vi "Autonomous Independent.vi"() -> ()   [LabVIEW 2014]
doc: "This VI is called when autonomous begins, and will automatically be terminated when autonomous ends. You can carry out timed or sensor driven robot movement independently without needing to return to the caller."
uses:
  <vilib>/Rock Robotics/WPI/SafetyOutput/WPI_SafetyOutputConfigMenu.ctl
  <vilib>/Rock Robotics/WPI/Joystick/WPI_JoystickGetSetRefNum.vi
  <vilib>/Rock Robotics/Network Tables/SD Read Boolean.vi
  <vilib>/Rock Robotics/Network Tables/SD Write Boolean.vi
  AutoVar.vi
  <vilib>/Rock Robotics/WPI/RobotDrive/WPI_RobotDriveGetSetRefNum.vi
  Global 2.vi
  <vilib>/Rock Robotics/WPI/RobotDrive/WPI_RobotDriveArcadeDrive_Standard(NoSaturation).vi
panel:
  out "Boolean1 2":bool
  out "Boolean1 3":bool
  out "Boolean1":bool
  out "Current Movement, for debugging":T1 {"Y Joystick Value" scale=1.0..-1.0; "X Joystick Value" scale=-1.0..1.0}
  in  "Array of robot movements":T2(array[cluster]) {"Y Joystick Value" scale=1.0..-1.0; "X Joystick Value" scale=-1.0..1.0}
  # "Be sure to right-click and choose Data Operations>>Make Current Value default if you want to save the array values with the VI"
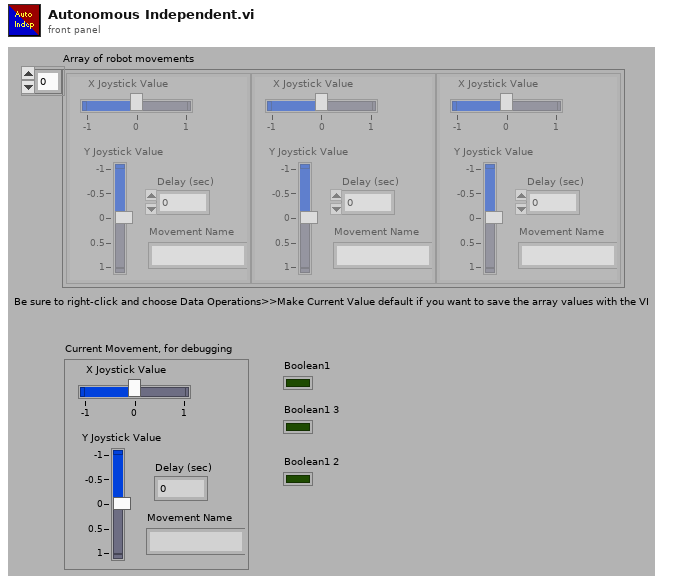
[diagram p1: front panel]
types:
  T1 = cluster{"X Joystick Value":dbl, "Y Joystick Value":dbl, "Delay (sec)":dbl, "Movement Name":string}
  T2 = cluster{"X Joystick Value":dbl, "Y Joystick Value":dbl, "Delay (sec)":dbl, "Movement Name":string}[]
  T3 = typedef "WPI_SafetyOutputConfigMenu.ctl" = enum16{"Enable", "Disable"}
  T4 = typedef "WPI_MotorControlDeviceRef.ctl" = cluster{"DeviceStatus":errorcluster, "Type":T5, "PWM":cluster{"Controller":T6, "PWM Channel":T7, "DeadBand":T8}, "CAN":cluster{"Device Number":u8, "Control Mode":T9, "Semaphore":T10, "Max Vout":dbl, "TalonSRX Control Mode":T11}, "Invert":bool, "TransformRef":T12, "InvTransformRef":T12}
  T5 = typedef "WPI_MotorControlType.ctl" = enum16{"PWM", "CAN", "CANTalonSRX"}
  T6 = typedef "FPGA_TypedefDigitalModule.ctl" = enum16{"Controller 1"}
  T7 = typedef "FPGA_DIOPWMChannel.ctl" = enum8{"PWM 0", "PWM 1", "PWM 2", "PWM 3", "PWM 4", "PWM 5", "PWM 6", "PWM 7", "PWM 8", "PWM 9", "PWM MXP 0", "PWM MXP 1", "PWM MXP 2", "PWM MXP 3", "PWM MXP 4", "PWM MXP 5", "PWM MXP 6", "PWM MXP 7", "PWM MXP 8", "PWM MXP 9", "Invalid"}
  T8 = typedef "WPI_PWMDeadband.ctl" = cluster{"Name":string, "maxPositivePwm":i32, "minPositivePwm":i32, "centerPwm":i32, "maxNegativePwm":i32, "minNegativePwm":i32, "angularRange":u16}
  T9 = typedef "WPI_CANJaguar_ControlMode.ctl" = enum8{"Percent VBus", "Current", "Speed", "Position", "Voltage"}
  T10 = typedef "Semaphore RefNum" = refnum<k1>
  T11 = typedef "WPI_CANTalonSRX_APIControlMode.ctl" = enum8{"Percent VBus", "Speed", "Position", "Slave", "Unchanged / Invalid"}
  T12 = typedef "WPI_PWMTransform_ConPane.ctl" = refnum<vi>
  T13 = typedef "WPI_RobotDriveDevRef.ctl" = cluster{"DevStatus":errorcluster, "Motors[]":T4[], "Square Inputs":bool, "Max Output":dbl}
  T14 = typedef "WPI_JoystickDevRef.ctl" = cluster{"Device":T15}
  T15 = typedef "WPI_JoystickDeviceEnum.ctl" = enum16{"USB 0", "USB 1", "USB 2", "USB 3", "USB 4", "USB 5"}
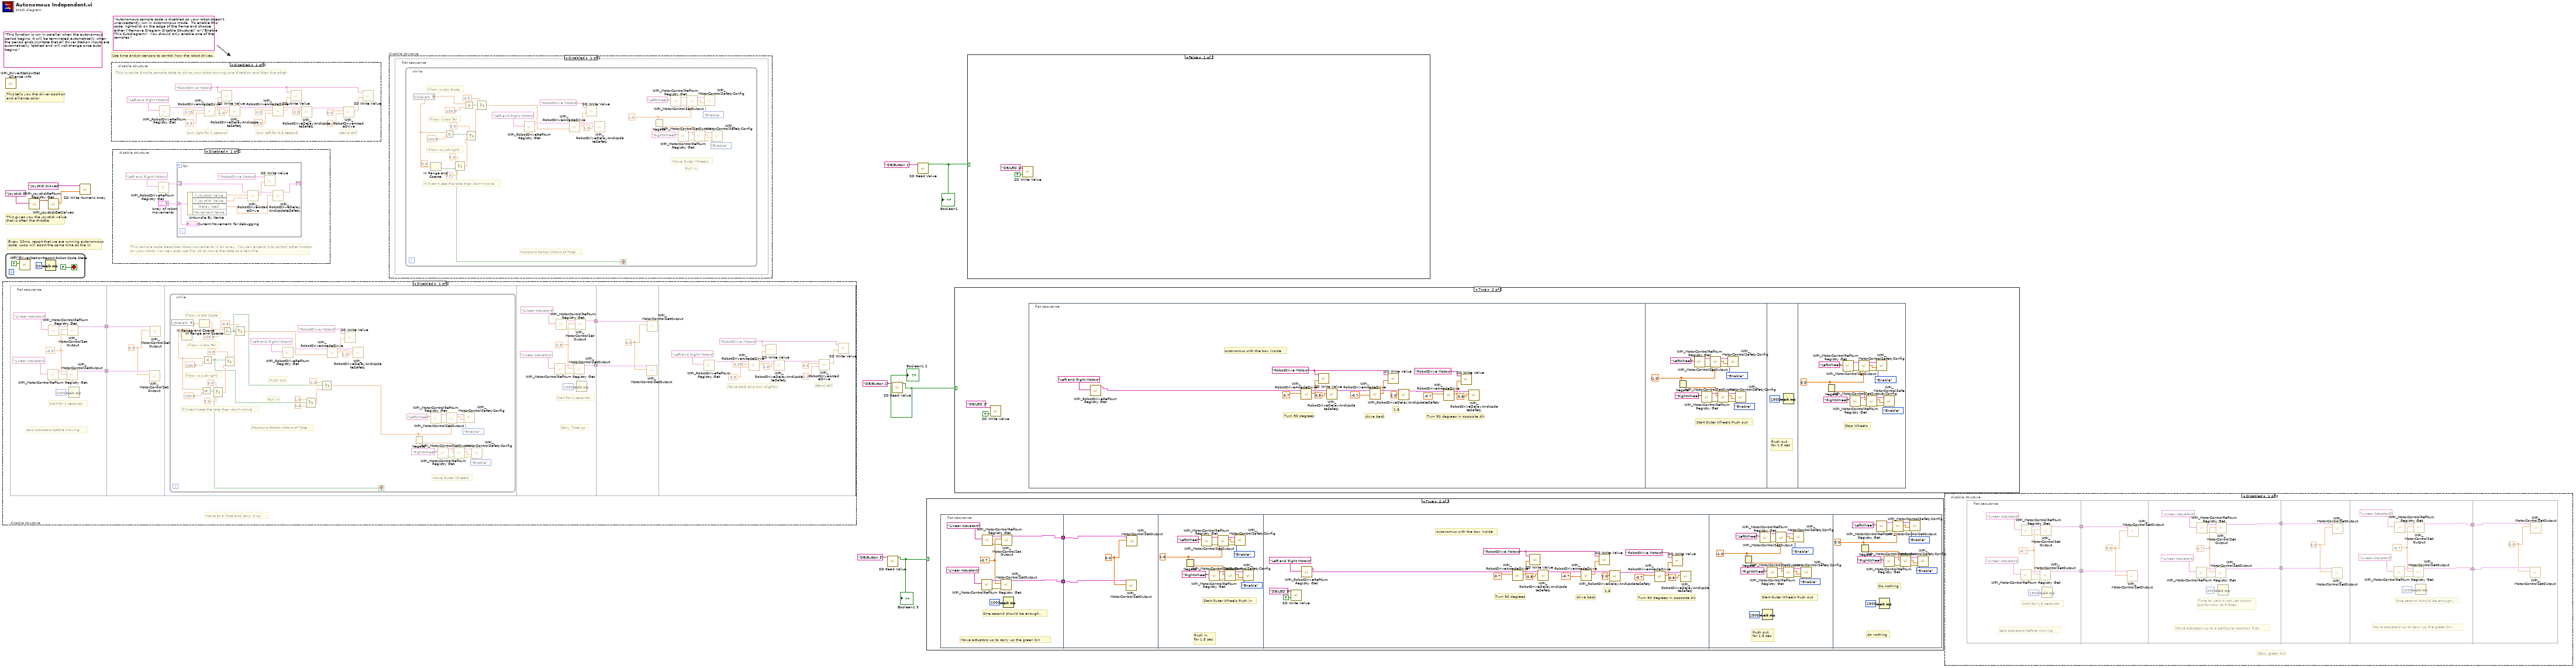
[diagram p0: block diagram]
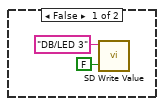
[diagram p3: hidden frame]
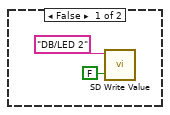
[diagram p4: hidden frame]
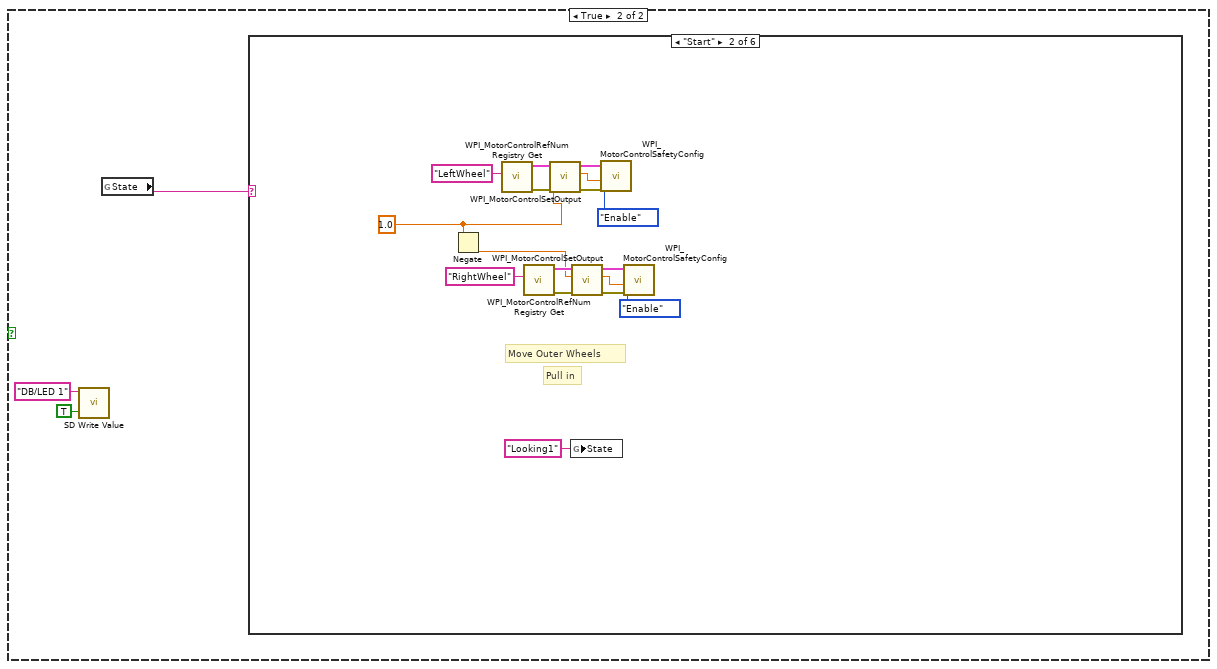
[diagram p5: hidden frame]
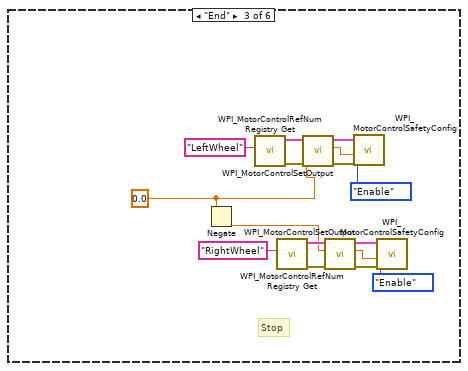
[diagram p7: hidden frame]
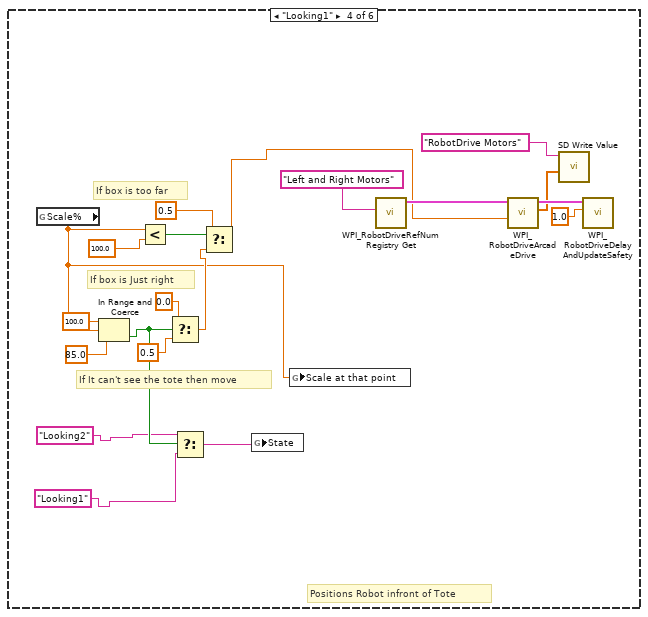
[diagram p8: hidden frame]
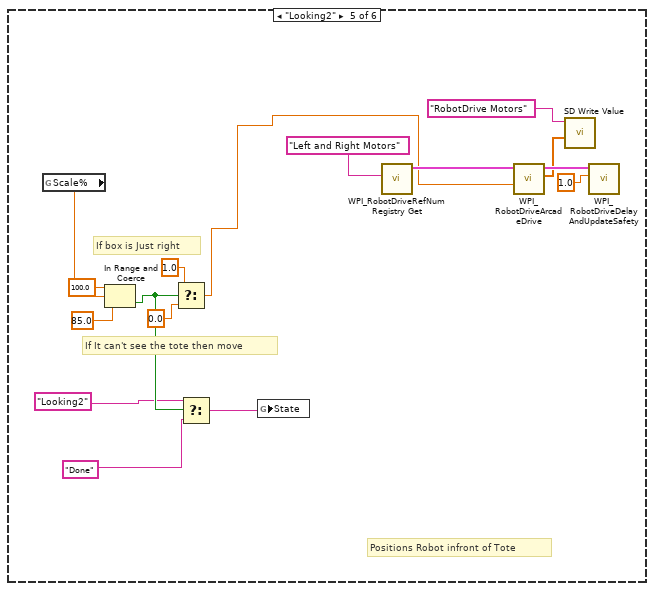
[diagram p9: hidden frame]
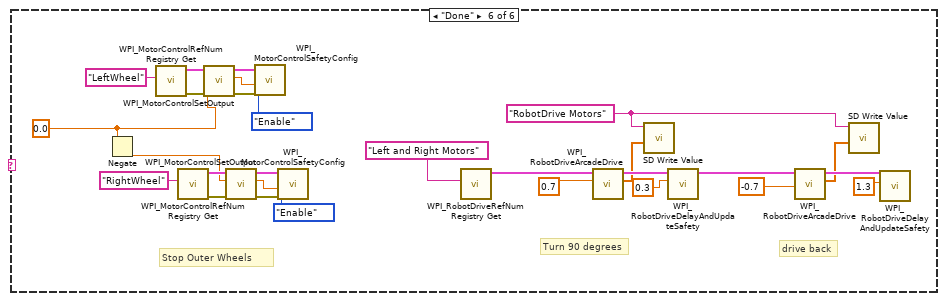
[diagram p10: hidden frame]
diagram:
  (unwired) "Autonomous sample code is disabled so your robot doesn't unexpectantly run in Autonomous mode.  To enable this code, right-click on the edge of the frame and choose either \"Remove Diagram Disable Structure\" or \"Enable This Subdiagram\". You should only enable one of the samples."
  (unwired) "This function is run in parallel when the autonomous period begins. It will be terminated automatically when the period ends.\n\nNote that all Driver Station inputs are automatically latched and will not change once auto begins."
  # "Every 20ms, report that we are running autonomous\ncode. Loop will abort the same time as the VI."
  # "This gives you the joystick value\nthat is often the throttle"
  # "Use time and/or sensors to control how the robot drives."
  # "This tells you the driver position\nand alliance color"
  n1 = disable-structure shown="Disabled" {
    frame Disabled {
      # "Move to a Tote and carry it up"
      n2 = flat-sequence {
        tunnel: [w16] -> w14
        tunnel: [w15] -> w13
        tunnel: w14 -> [w27]
        tunnel: w13 -> [w26]
        tunnel: [w71] -> w12
        tunnel: [w70] -> w11
        tunnel: w12 -> [w81]
        tunnel: w11 -> [w80]
        frame #0 {
          w18 = -0.5 ("Output")
          # "zero actuators before moving"
          # "Wait for 1 seconds"
          n3 = call <vilib>:"WPI_MotorControlRefNum Registry Get.vi"("refnum name"="Linear Actuator1") -> ("error out"=w21:errorcluster, "MotorControlDevRef"=w20:T4)  [unwired: 9 in]
          n4 = call <vilib>:"WPI_MotorControlRefNum Registry Get.vi"("refnum name"="Linear Actuator0") -> ("error out"=w24:errorcluster, "MotorControlDevRef"=w23:T4)  [unwired: 9 in]
          n5 = call <vilib>:"WPI_MotorControlSetOutput.vi"("error in (no error)"=w21, "Output"=w18, "MotorControlDevRef"=w20) -> ("MotorControlDevRef"=w15:T4)  [unwired: 6 in, 2 out]
          n6 = call <vilib>:"WPI_MotorControlSetOutput.vi"("error in (no error)"=w24, "Output"=w18, "MotorControlDevRef"=w23) -> ("MotorControlDevRef"=w16:T4)  [unwired: 6 in, 2 out]
          n7 = Wait (ms)(milliseconds to wait=u32 1000) -> ()  [unwired: 1 out]
        }
        frame #1 {
          w25 = 0.0 ("Output")
          n8 = call <vilib>:"WPI_MotorControlSetOutput.vi"("Output"=w25, "MotorControlDevRef"=w26) -> ()  [unwired: 7 in, 3 out]
          n9 = call <vilib>:"WPI_MotorControlSetOutput.vi"("Output"=w25, "MotorControlDevRef"=w27) -> ()  [unwired: 7 in, 3 out]
        }
        frame #2 {
          n10 = while {
            stop <- w54 stop-if-true
            # "Move Outer Wheels"
            # "Pull in"
            # "Push out"
            # "If It can't see the tote then don't move"
            # "Positions Robot infront of Tote"
            # "If box is Just right"
            # "If box is too Far"
            # "If box is too close"
            n11 = global read "Global 2.vi" "Scale%"() -> (w29:dbl)
            n12 = In Range and Coerce(x=w29) -> (coerced(x)=w28:dbl)  [unwired: 2 in, 1 out]
            n13 = In Range and Coerce(x=w29) -> (coerced(x)=w30:dbl)  [unwired: 2 in, 1 out]
            n14 = Equal?(x=w28, y=100.0) -> (x = y?=w54:bool)
            n15 = Less?(x=w28, y=100.0) -> (x < y?=w33:bool)
            n16 = Select(t=0.0, s=w54, f=0.0) -> (s? t:f=w62:dbl)
            n17 = Greater?(x=w30, y=100.0) -> (0:w38:bool)
            n18 = Select(t=0.5, s=w33, f=w62) -> (s? t:f=w65:dbl)
            n19 = Select(t=-0.5, s=w38, f=w65) -> (s? t:f=w55:dbl)
            n20 = call <vilib>:"WPI_RobotDriveRefNum Registry Get.vi"("refnum name"="Left and Right Motors") -> ("RobotDriveDevRef"=w58:T13)  [unwired: 1 in, 9 out]
            n21 = Select(t=1.0, s=w33, f=0.0) -> (s? t:f=w34:dbl)
            n22 = Select(t=-1.0, s=w38, f=w34) -> (s? t:f=w36:dbl)
            n23 = call-poly <vilib>:"WPI_RobotDriveArcadeDrive.vi"("Y axis value"=w55, "RobotDriveDevRef"=w58) -> ("Motor Values"=w57:dbl[], "RobotDriveDevRef"=w61:T13)  [unwired: 2 in, 6 out]
            n24 = call-poly <vilib>:"SD Write Value.vi"("Numeric Array"=w57, "Name"="RobotDrive Motors") -> ()  [unwired: 8 in, 2 out]
            n25 = call <vilib>:"WPI_RobotDriveDelayAndUpdateSafety.vi"("Delay (s)"=1.0, "RobotDriveDevRef"=w61) -> ()  [unwired: 8 in, 2 out]
            n26 = Negate(x=w36) -> (-x=w35:dbl)
            n27 = call <vilib>:"WPI_MotorControlRefNum Registry Get.vi"("refnum name"="LeftWheel") -> ("error out"=w52:errorcluster, "MotorControlDevRef"=w51:T4)  [unwired: 9 in]
            n28 = call <vilib>:"WPI_MotorControlRefNum Registry Get.vi"("refnum name"="RightWheel") -> ("error out"=w50:errorcluster, "MotorControlDevRef"=w49:T4)  [unwired: 9 in]
            n29 = call <vilib>:"WPI_MotorControlSetOutput.vi"("error in (no error)"=w52, "Output"=w36, "MotorControlDevRef"=w51) -> ("error out"=w46:errorcluster, "Motor Output"=w45:dbl, "MotorControlDevRef"=w44:T4)  [unwired: 6 in]
            n30 = call <vilib>:"WPI_MotorControlSetOutput.vi"("error in (no error)"=w50, "Output"=w35, "MotorControlDevRef"=w49) -> ("error out"=w43:errorcluster, "Motor Output"=w42:dbl, "MotorControlDevRef"=w41:T4)  [unwired: 6 in]
            n31 = call <vilib>:"WPI_MotorControlSafetyConfig.vi"("error in (no error)"=w46, "timeout (s)"=w45, "mode"=WPI_SafetyOutputConfigMenu."Enable", "MotorControlDevRef"=w44) -> ()  [unwired: 6 in, 2 out]
            n32 = call <vilib>:"WPI_MotorControlSafetyConfig.vi"("error in (no error)"=w43, "timeout (s)"=w42, "mode"=WPI_SafetyOutputConfigMenu."Enable", "MotorControlDevRef"=w41) -> ()  [unwired: 6 in, 2 out]
          }
        }
        frame #3 {
          w73 = 0.5 ("Output")
          # "Carry Tote up"
          # "Wait for 1 seconds"
          n33 = call <vilib>:"WPI_MotorControlRefNum Registry Get.vi"("refnum name"="Linear Actuator1") -> ("error out"=w76:errorcluster, "MotorControlDevRef"=w75:T4)  [unwired: 9 in]
          n34 = call <vilib>:"WPI_MotorControlRefNum Registry Get.vi"("refnum name"="Linear Actuator0") -> ("error out"=w79:errorcluster, "MotorControlDevRef"=w78:T4)  [unwired: 9 in]
          n35 = call <vilib>:"WPI_MotorControlSetOutput.vi"("error in (no error)"=w76, "Output"=w73, "MotorControlDevRef"=w75) -> ("MotorControlDevRef"=w70:T4)  [unwired: 6 in, 2 out]
          n36 = call <vilib>:"WPI_MotorControlSetOutput.vi"("error in (no error)"=w79, "Output"=w73, "MotorControlDevRef"=w78) -> ("MotorControlDevRef"=w71:T4)  [unwired: 6 in, 2 out]
          n37 = Wait (ms)(milliseconds to wait=u32 1000) -> ()  [unwired: 1 out]
        }
        frame #4 {
          w82 = 0.0 ("Output")
          n38 = call <vilib>:"WPI_MotorControlSetOutput.vi"("Output"=w82, "MotorControlDevRef"=w80) -> ()  [unwired: 7 in, 3 out]
          n39 = call <vilib>:"WPI_MotorControlSetOutput.vi"("Output"=w82, "MotorControlDevRef"=w81) -> ()  [unwired: 7 in, 3 out]
        }
        frame #5 {
          w83 = "RobotDrive Motors" ("Name")
          # "stand still"
          # "Move back and turn slightly"
          n40 = call <vilib>:"WPI_RobotDriveRefNum Registry Get.vi"("refnum name"="Left and Right Motors") -> ("RobotDriveDevRef"=w90:T13)  [unwired: 1 in, 9 out]
          n41 = call-poly <vilib>:"WPI_RobotDriveArcadeDrive.vi"("Y axis value"=-0.5 ("X axis value"), "X axis value"=0.25, "RobotDriveDevRef"=w90) -> ("Motor Values"=w89:dbl[], "RobotDriveDevRef"=w93:T13)  [unwired: 1 in, 6 out]
          n42 = call-poly <vilib>:"SD Write Value.vi"("Numeric Array"=w89, "Name"=w83) -> ()  [unwired: 8 in, 2 out]
          n43 = call <vilib>:"WPI_RobotDriveDelayAndUpdateSafety.vi"("Delay (s)"=2.0, "RobotDriveDevRef"=w93) -> ("RobotDriveDevRef 2"=w84:T13)  [unwired: 8 in, 1 out]
          n44 = call-poly <vilib>:"WPI_RobotDriveArcadeDrive.vi"("Y axis value"=0.0 ("X axis value"), "X axis value"=0.0, "RobotDriveDevRef"=w84) -> ("Motor Values"=w85:dbl[])  [unwired: 1 in, 7 out]
          n45 = call-poly <vilib>:"SD Write Value.vi"("Numeric Array"=w85, "Name"=w83) -> ()  [unwired: 8 in, 2 out]
        }
      }
    }
    frame Enabled {
    }
  }
  n46 = while {
    stop <- FALSE stop-if-true
    n47 = call <vilib>:"WPI_DriverStationReport Robot Code State.vi"("Autonomous"=TRUE) -> ()  [unwired: 10 in, 1 out]
    n48 = Wait (ms)(milliseconds to wait=u32 20) -> ()  [unwired: 1 out]
  }
  n49 = call <vilib>:"WPI_DriverStationGet Alliance Info.vi"() -> ()  [unwired: 12 out]
  n50 = call <vilib>:"WPI_JoystickRefNum Registry Get.vi"("refnum name"="Joystick 0") -> ("JoystickDevRef"=w9:T14)  [unwired: 1 in, 9 out]
  n51 = call <vilib>:"WPI_JoystickGetValues.vi"("JoystickDevRef"=w9) -> ("Axes"=w7:dbl[])  [unwired: 6 in, 4 out]
  n52 = call <vilib>:"SD Write Numeric Array.vi"("Numeric Array"=w7, "Name"="Joystick 0/Axes") -> ()  [unwired: 8 in, 2 out]
  n53 = disable-structure shown="Disabled" {
    frame Disabled {
      w98 = "RobotDrive Motors" ("Name")
      # "This is some simple sample code to drive your robot curving one direction and then the other."
      # "stand still"
      # "turn left for 0.5 second"
      # "turn right for 1 second"
      n54 = call <vilib>:"WPI_RobotDriveRefNum Registry Get.vi"("refnum name"="Left and Right Motors") -> ("RobotDriveDevRef"=w102:T13)  [unwired: 1 in, 9 out]
      n55 = call-poly <vilib>:"WPI_RobotDriveArcadeDrive.vi"("Y axis value"=0.5 ("X axis value"), "X axis value"=0.25, "RobotDriveDevRef"=w102) -> ("Motor Values"=w101:dbl[], "RobotDriveDevRef"=w109:T13)  [unwired: 1 in, 6 out]
      n56 = call-poly <vilib>:"SD Write Value.vi"("Numeric Array"=w101, "Name"=w98) -> ()  [unwired: 8 in, 2 out]
      n57 = call <vilib>:"WPI_RobotDriveDelayAndUpdateSafety.vi"("Delay (s)"=1.0, "RobotDriveDevRef"=w109) -> ("RobotDriveDevRef 2"=w108:T13)  [unwired: 8 in, 1 out]
      n58 = call-poly <vilib>:"WPI_RobotDriveArcadeDrive.vi"("Y axis value"=0.25 ("X axis value"), "X axis value"=0.5, "RobotDriveDevRef"=w108) -> ("Motor Values"=w100:dbl[], "RobotDriveDevRef"=w107:T13)  [unwired: 1 in, 6 out]
      n59 = call-poly <vilib>:"SD Write Value.vi"("Numeric Array"=w100, "Name"=w98) -> ()  [unwired: 8 in, 2 out]
      n60 = call <vilib>:"WPI_RobotDriveDelayAndUpdateSafety.vi"("Delay (s)"=0.5, "RobotDriveDevRef"=w107) -> ("RobotDriveDevRef 2"=w106:T13)  [unwired: 8 in, 1 out]
      n61 = call-poly <vilib>:"WPI_RobotDriveArcadeDrive.vi"("Y axis value"=0.0 ("X axis value"), "X axis value"=0.0, "RobotDriveDevRef"=w106) -> ("Motor Values"=w99:dbl[])  [unwired: 1 in, 7 out]
      n62 = call-poly <vilib>:"SD Write Value.vi"("Numeric Array"=w99, "Name"=w98) -> ()  [unwired: 8 in, 2 out]
    }
    frame Enabled {
    }
  }
  n63 = disable-structure shown="Disabled" {
    frame Disabled {
      # "This sample code describes robot movements in an array. You can extend it to control other motors\non your robot. You can also use file I/O to move the data to a text file."
      n64 = call <vilib>:"WPI_RobotDriveRefNum Registry Get.vi"("refnum name"="Left and Right Motors") -> ("RobotDriveDevRef"=w117:T13)  [unwired: 1 in, 9 out]
      n65 = for {
        shift-right: [w125] -> _
        shift-left: w117 -> [w126]
        tunnel: "Array of robot movements" -> [w121] mode=indexing
        n66 = Unbundle By Name(w121) -> ("X Joystick Value"=w124:dbl, "Y Joystick Value"=w123:dbl, "Delay (sec)"=w122:dbl)  [unwired: 1 out]
        n67 = call-poly <vilib>:"WPI_RobotDriveArcadeDrive.vi"("Y axis value"=w123, "X axis value"=w124, "RobotDriveDevRef"=w126) -> ("Motor Values"=w119:dbl[], "RobotDriveDevRef"=w127:T13)  [unwired: 1 in, 6 out]
        n68 = call-poly <vilib>:"SD Write Value.vi"("Numeric Array"=w119, "Name"="RobotDrive Motors") -> ()  [unwired: 8 in, 2 out]
        n69 = call <vilib>:"WPI_RobotDriveDelayAndUpdateSafety.vi"("Delay (s)"=w122, "RobotDriveDevRef"=w127) -> ("RobotDriveDevRef 2"=w125:T13)  [unwired: 8 in, 1 out]
        "Current Movement, for debugging" <- w121
      }
    }
    frame Enabled {
    }
  }
  n70 = disable-structure shown="Disabled" {
    frame Disabled {
      n71 = flat-sequence {
        frame #0 {
          n72 = while {
            stop <- w131 stop-if-true
            w128 = 1.0 ("t")
            # "Move Outer Wheels"
            # "Pull in"
            # "If It can't see the tote then don't move"
            # "Positions Robot infront of Tote"
            # "If box is Just right"
            # "If box is too far"
            # "If box is too close"
            n73 = global read "Global 2.vi" "Scale%"() -> (w130:dbl)
            n74 = In Range and Coerce(upper limit=0.0, x=w130) -> (In Range?=w131:bool)  [unwired: 1 in, 1 out]
            n75 = Less?(x=w130, y=100.0) -> (x < y?=w132:bool)
            n76 = Select(t=0.0, s=w131, f=0.0) -> (s? t:f=w157:dbl)
            n77 = Greater?(x=w130, y=100.0) -> (0:w134:bool)
            n78 = Select(t=0.5, s=w132, f=w157) -> (s? t:f=w159:dbl)
            n79 = Select(t=-0.5, s=w134, f=w159) -> (s? t:f=w150:dbl)
            n80 = call <vilib>:"WPI_RobotDriveRefNum Registry Get.vi"("refnum name"="Left and Right Motors") -> ("RobotDriveDevRef"=w153:T13)  [unwired: 1 in, 9 out]
            n81 = call-poly <vilib>:"WPI_RobotDriveArcadeDrive.vi"("Y axis value"=w150, "RobotDriveDevRef"=w153) -> ("Motor Values"=w152:dbl[], "RobotDriveDevRef"=w156:T13)  [unwired: 2 in, 6 out]
            n82 = call-poly <vilib>:"SD Write Value.vi"("Numeric Array"=w152, "Name"="RobotDrive Motors") -> ()  [unwired: 8 in, 2 out]
            n83 = call <vilib>:"WPI_RobotDriveDelayAndUpdateSafety.vi"("Delay (s)"=1.0, "RobotDriveDevRef"=w156) -> ()  [unwired: 8 in, 2 out]
            n84 = Negate(x=w128) -> (-x=w133:dbl)
            n85 = call <vilib>:"WPI_MotorControlRefNum Registry Get.vi"("refnum name"="LeftWheel") -> ("error out"=w148:errorcluster, "MotorControlDevRef"=w147:T4)  [unwired: 9 in]
            n86 = call <vilib>:"WPI_MotorControlRefNum Registry Get.vi"("refnum name"="RightWheel") -> ("error out"=w146:errorcluster, "MotorControlDevRef"=w145:T4)  [unwired: 9 in]
            n87 = call <vilib>:"WPI_MotorControlSetOutput.vi"("error in (no error)"=w148, "Output"=w128, "MotorControlDevRef"=w147) -> ("error out"=w142:errorcluster, "Motor Output"=w141:dbl, "MotorControlDevRef"=w140:T4)  [unwired: 6 in]
            n88 = call <vilib>:"WPI_MotorControlSetOutput.vi"("error in (no error)"=w146, "Output"=w133, "MotorControlDevRef"=w145) -> ("error out"=w139:errorcluster, "Motor Output"=w138:dbl, "MotorControlDevRef"=w137:T4)  [unwired: 6 in]
            n89 = call <vilib>:"WPI_MotorControlSafetyConfig.vi"("error in (no error)"=w142, "timeout (s)"=w141, "mode"=WPI_SafetyOutputConfigMenu."Enable", "MotorControlDevRef"=w140) -> ()  [unwired: 6 in, 2 out]
            n90 = call <vilib>:"WPI_MotorControlSafetyConfig.vi"("error in (no error)"=w139, "timeout (s)"=w138, "mode"=WPI_SafetyOutputConfigMenu."Enable", "MotorControlDevRef"=w137) -> ()  [unwired: 6 in, 2 out]
          }
        }
      }
    }
    frame Enabled {
    }
  }
  n91 = call-poly <vilib>:"SD Read Value.vi"("Name"="DB/Button 3") -> ("Boolean"=w2:bool)  [unwired: 8 in, 2 out]
  "Boolean1 3" <- w2
  n92 = call-poly <vilib>:"SD Read Value.vi"("Name"="DB/Button 2") -> ("Boolean"=w1:bool)  [unwired: 8 in, 2 out]
  "Boolean1 2" <- w1
  n93 = call-poly <vilib>:"SD Read Value.vi"("Name"="DB/Button 1") -> ("Boolean"=w3:bool)  [unwired: 8 in, 2 out]
  "Boolean1" <- w3
  n94 = case shown="True" w2 {
    frame False {
      n95 = call-poly <vilib>:"SD Write Value.vi"("Boolean"=FALSE, "Name"="DB/LED 3") -> ()  [unwired: 8 in, 2 out]
    }
    frame True {
      n96 = flat-sequence {
        tunnel: [w169] -> w167
        tunnel: [w168] -> w166
        tunnel: w167 -> [w179]
        tunnel: w166 -> [w178]
        frame #0 {
          w171 = -0.7 ("Output")
          # "Move actuators up to carry up the green bin"
          # "One second should be enough.."
          n97 = call <vilib>:"WPI_MotorControlRefNum Registry Get.vi"("refnum name"="Linear Actuator1") -> ("error out"=w174:errorcluster, "MotorControlDevRef"=w173:T4)  [unwired: 9 in]
          n98 = call <vilib>:"WPI_MotorControlRefNum Registry Get.vi"("refnum name"="Linear Actuator0") -> ("error out"=w177:errorcluster, "MotorControlDevRef"=w176:T4)  [unwired: 9 in]
          n99 = call <vilib>:"WPI_MotorControlSetOutput.vi"("error in (no error)"=w174, "Output"=w171, "MotorControlDevRef"=w173) -> ("MotorControlDevRef"=w169:T4)  [unwired: 6 in, 2 out]
          n100 = call <vilib>:"WPI_MotorControlSetOutput.vi"("error in (no error)"=w177, "Output"=w171, "MotorControlDevRef"=w176) -> ("MotorControlDevRef"=w168:T4)  [unwired: 6 in, 2 out]
          n101 = Wait (ms)(milliseconds to wait=u32 1000) -> ()  [unwired: 1 out]
        }
        frame #1 {
          w180 = 0.0 ("Output")
          n102 = call <vilib>:"WPI_MotorControlSetOutput.vi"("Output"=w180, "MotorControlDevRef"=w179) -> ()  [unwired: 7 in, 3 out]
          n103 = call <vilib>:"WPI_MotorControlSetOutput.vi"("Output"=w180, "MotorControlDevRef"=w178) -> ()  [unwired: 7 in, 3 out]
        }
        frame #2 {
          w181 = 1.0 ("t")
          # "Push in \nfor 1.5 sec"
          # "Start Outer Wheels Push in"
          n104 = Negate(x=w181) -> (-x=w182:dbl)
          n105 = call <vilib>:"WPI_MotorControlRefNum Registry Get.vi"("refnum name"="LeftWheel") -> ("error out"=w196:errorcluster, "MotorControlDevRef"=w195:T4)  [unwired: 9 in]
          n106 = call <vilib>:"WPI_MotorControlRefNum Registry Get.vi"("refnum name"="RightWheel") -> ("error out"=w194:errorcluster, "MotorControlDevRef"=w193:T4)  [unwired: 9 in]
          n107 = call <vilib>:"WPI_MotorControlSetOutput.vi"("error in (no error)"=w196, "Output"=w181, "MotorControlDevRef"=w195) -> ("error out"=w190:errorcluster, "Motor Output"=w189:dbl, "MotorControlDevRef"=w188:T4)  [unwired: 6 in]
          n108 = call <vilib>:"WPI_MotorControlSetOutput.vi"("error in (no error)"=w194, "Output"=w182, "MotorControlDevRef"=w193) -> ("error out"=w187:errorcluster, "Motor Output"=w186:dbl, "MotorControlDevRef"=w185:T4)  [unwired: 6 in]
          n109 = call <vilib>:"WPI_MotorControlSafetyConfig.vi"("error in (no error)"=w190, "timeout (s)"=w189, "mode"=WPI_SafetyOutputConfigMenu."Enable", "MotorControlDevRef"=w188) -> ()  [unwired: 6 in, 2 out]
          n110 = call <vilib>:"WPI_MotorControlSafetyConfig.vi"("error in (no error)"=w187, "timeout (s)"=w186, "mode"=WPI_SafetyOutputConfigMenu."Enable", "MotorControlDevRef"=w185) -> ()  [unwired: 6 in, 2 out]
        }
        frame #3 {
          w207 = "RobotDrive Motors" ("Name")
          # "1.6"
          # "Autonomus with the box inside"
          # "Turn 90 degrees in opposite dir."
          # "drive back"
          # "Turn 90 degrees"
          n111 = call-poly <vilib>:"SD Write Value.vi"("Boolean"=TRUE, "Name"="DB/LED 3") -> ()  [unwired: 8 in, 2 out]
          n112 = call <vilib>:"WPI_RobotDriveRefNum Registry Get.vi"("refnum name"="Left and Right Motors") -> ("RobotDriveDevRef"=w197:T13)  [unwired: 1 in, 9 out]
          n113 = call-poly <vilib>:"WPI_RobotDriveArcadeDrive.vi"("X axis value"=0.7, "RobotDriveDevRef"=w197) -> ("Motor Values"=w209:dbl[], "RobotDriveDevRef"=w215:T13)  [unwired: 2 in, 6 out]
          n114 = call-poly <vilib>:"SD Write Value.vi"("Numeric Array"=w209, "Name"=w207) -> ()  [unwired: 8 in, 2 out]
          n115 = call <vilib>:"WPI_RobotDriveDelayAndUpdateSafety.vi"("Delay (s)"=0.8, "RobotDriveDevRef"=w215) -> ("RobotDriveDevRef 2"=w214:T13)  [unwired: 8 in, 1 out]
          n116 = call-poly <vilib>:"WPI_RobotDriveArcadeDrive.vi"("Y axis value"=-0.7 ("X axis value"), "RobotDriveDevRef"=w214) -> ("Motor Values"=w208:dbl[], "RobotDriveDevRef"=w213:T13)  [unwired: 2 in, 6 out]
          n117 = call-poly <vilib>:"SD Write Value.vi"("Numeric Array"=w208, "Name"=w207) -> ()  [unwired: 8 in, 2 out]
          n118 = call <vilib>:"WPI_RobotDriveDelayAndUpdateSafety.vi"("Delay (s)"=2.0, "RobotDriveDevRef"=w213) -> ("RobotDriveDevRef 2"=w200:T13)  [unwired: 8 in, 1 out]
          n119 = call-poly <vilib>:"WPI_RobotDriveArcadeDrive.vi"("X axis value"=-0.7, "RobotDriveDevRef"=w200) -> ("Motor Values"=w202:dbl[], "RobotDriveDevRef"=w204:T13)  [unwired: 2 in, 6 out]
          n120 = call-poly <vilib>:"SD Write Value.vi"("Numeric Array"=w202, "Name"="RobotDrive Motors") -> ()  [unwired: 8 in, 2 out]
          n121 = call <vilib>:"WPI_RobotDriveDelayAndUpdateSafety.vi"("Delay (s)"=0.8, "RobotDriveDevRef"=w204) -> ()  [unwired: 8 in, 2 out]
        }
        frame #4 {
          w218 = -1.0 ("t")
          # "Push out \nfor 1.5 sec"
          # "Start Outer Wheels Push out"
          n122 = Negate(x=w218) -> (-x=w219:dbl)
          n123 = call <vilib>:"WPI_MotorControlRefNum Registry Get.vi"("refnum name"="LeftWheel") -> ("error out"=w233:errorcluster, "MotorControlDevRef"=w232:T4)  [unwired: 9 in]
          n124 = Wait (ms)(milliseconds to wait=u32 1500) -> ()  [unwired: 1 out]
          n125 = call <vilib>:"WPI_MotorControlRefNum Registry Get.vi"("refnum name"="RightWheel") -> ("error out"=w231:errorcluster, "MotorControlDevRef"=w230:T4)  [unwired: 9 in]
          n126 = call <vilib>:"WPI_MotorControlSetOutput.vi"("error in (no error)"=w233, "Output"=w218, "MotorControlDevRef"=w232) -> ("error out"=w227:errorcluster, "Motor Output"=w226:dbl, "MotorControlDevRef"=w225:T4)  [unwired: 6 in]
          n127 = call <vilib>:"WPI_MotorControlSetOutput.vi"("error in (no error)"=w231, "Output"=w219, "MotorControlDevRef"=w230) -> ("error out"=w224:errorcluster, "Motor Output"=w223:dbl, "MotorControlDevRef"=w222:T4)  [unwired: 6 in]
          n128 = call <vilib>:"WPI_MotorControlSafetyConfig.vi"("error in (no error)"=w227, "timeout (s)"=w226, "mode"=WPI_SafetyOutputConfigMenu."Enable", "MotorControlDevRef"=w225) -> ()  [unwired: 6 in, 2 out]
          n129 = call <vilib>:"WPI_MotorControlSafetyConfig.vi"("error in (no error)"=w224, "timeout (s)"=w223, "mode"=WPI_SafetyOutputConfigMenu."Enable", "MotorControlDevRef"=w222) -> ()  [unwired: 6 in, 2 out]
        }
        frame #5 {
          w235 = 0.0 ("t")
          # "do nothing"
          # "Do nothing"
          n130 = Negate(x=w235) -> (-x=w236:dbl)
          n131 = call <vilib>:"WPI_MotorControlRefNum Registry Get.vi"("refnum name"="LeftWheel") -> ("error out"=w250:errorcluster, "MotorControlDevRef"=w249:T4)  [unwired: 9 in]
          n132 = Wait (ms)(milliseconds to wait=u32 1500) -> ()  [unwired: 1 out]
          n133 = call <vilib>:"WPI_MotorControlRefNum Registry Get.vi"("refnum name"="RightWheel") -> ("error out"=w248:errorcluster, "MotorControlDevRef"=w247:T4)  [unwired: 9 in]
          n134 = call <vilib>:"WPI_MotorControlSetOutput.vi"("error in (no error)"=w250, "Output"=w235, "MotorControlDevRef"=w249) -> ("error out"=w244:errorcluster, "Motor Output"=w243:dbl, "MotorControlDevRef"=w242:T4)  [unwired: 6 in]
          n135 = call <vilib>:"WPI_MotorControlSetOutput.vi"("error in (no error)"=w248, "Output"=w236, "MotorControlDevRef"=w247) -> ("error out"=w241:errorcluster, "Motor Output"=w240:dbl, "MotorControlDevRef"=w239:T4)  [unwired: 6 in]
          n136 = call <vilib>:"WPI_MotorControlSafetyConfig.vi"("error in (no error)"=w244, "timeout (s)"=w243, "mode"=WPI_SafetyOutputConfigMenu."Enable", "MotorControlDevRef"=w242) -> ()  [unwired: 6 in, 2 out]
          n137 = call <vilib>:"WPI_MotorControlSafetyConfig.vi"("error in (no error)"=w241, "timeout (s)"=w240, "mode"=WPI_SafetyOutputConfigMenu."Enable", "MotorControlDevRef"=w239) -> ()  [unwired: 6 in, 2 out]
        }
      }
    }
  }
  n138 = case shown="True" w1 {
    frame False {
      n139 = call-poly <vilib>:"SD Write Value.vi"("Boolean"=FALSE, "Name"="DB/LED 2") -> ()  [unwired: 8 in, 2 out]
    }
    frame True {
      n140 = call-poly <vilib>:"SD Write Value.vi"("Boolean"=TRUE, "Name"="DB/LED 2") -> ()  [unwired: 8 in, 2 out]
      n141 = flat-sequence {
        frame #0 {
          w263 = "RobotDrive Motors" ("Name")
          # "1.6"
          # "Autonomus with the box inside"
          # "Turn 90 degrees in opposite dir."
          # "drive back"
          # "Turn 90 degrees"
          n142 = call <vilib>:"WPI_RobotDriveRefNum Registry Get.vi"("refnum name"="Left and Right Motors") -> ("RobotDriveDevRef"=w255:T13)  [unwired: 1 in, 9 out]
          n143 = call-poly <vilib>:"WPI_RobotDriveArcadeDrive.vi"("X axis value"=0.7, "RobotDriveDevRef"=w255) -> ("Motor Values"=w265:dbl[], "RobotDriveDevRef"=w271:T13)  [unwired: 2 in, 6 out]
          n144 = call-poly <vilib>:"SD Write Value.vi"("Numeric Array"=w265, "Name"=w263) -> ()  [unwired: 8 in, 2 out]
          n145 = call <vilib>:"WPI_RobotDriveDelayAndUpdateSafety.vi"("Delay (s)"=0.8, "RobotDriveDevRef"=w271) -> ("RobotDriveDevRef 2"=w270:T13)  [unwired: 8 in, 1 out]
          n146 = call-poly <vilib>:"WPI_RobotDriveArcadeDrive.vi"("Y axis value"=-0.7 ("X axis value"), "RobotDriveDevRef"=w270) -> ("Motor Values"=w264:dbl[], "RobotDriveDevRef"=w269:T13)  [unwired: 2 in, 6 out]
          n147 = call-poly <vilib>:"SD Write Value.vi"("Numeric Array"=w264, "Name"=w263) -> ()  [unwired: 8 in, 2 out]
          n148 = call <vilib>:"WPI_RobotDriveDelayAndUpdateSafety.vi"("Delay (s)"=2.0, "RobotDriveDevRef"=w269) -> ("RobotDriveDevRef 2"=w256:T13)  [unwired: 8 in, 1 out]
          n149 = call-poly <vilib>:"WPI_RobotDriveArcadeDrive.vi"("X axis value"=-0.7, "RobotDriveDevRef"=w256) -> ("Motor Values"=w258:dbl[], "RobotDriveDevRef"=w260:T13)  [unwired: 2 in, 6 out]
          n150 = call-poly <vilib>:"SD Write Value.vi"("Numeric Array"=w258, "Name"="RobotDrive Motors") -> ()  [unwired: 8 in, 2 out]
          n151 = call <vilib>:"WPI_RobotDriveDelayAndUpdateSafety.vi"("Delay (s)"=0.8, "RobotDriveDevRef"=w260) -> ()  [unwired: 8 in, 2 out]
        }
        frame #1 {
          w273 = -1.0 ("t")
          # "Start Outer Wheels Push out"
          n152 = Negate(x=w273) -> (-x=w274:dbl)
          n153 = call <vilib>:"WPI_MotorControlRefNum Registry Get.vi"("refnum name"="LeftWheel") -> ("error out"=w288:errorcluster, "MotorControlDevRef"=w287:T4)  [unwired: 9 in]
          n154 = call <vilib>:"WPI_MotorControlRefNum Registry Get.vi"("refnum name"="RightWheel") -> ("error out"=w286:errorcluster, "MotorControlDevRef"=w285:T4)  [unwired: 9 in]
          n155 = call <vilib>:"WPI_MotorControlSetOutput.vi"("error in (no error)"=w288, "Output"=w273, "MotorControlDevRef"=w287) -> ("error out"=w282:errorcluster, "Motor Output"=w281:dbl, "MotorControlDevRef"=w280:T4)  [unwired: 6 in]
          n156 = call <vilib>:"WPI_MotorControlSetOutput.vi"("error in (no error)"=w286, "Output"=w274, "MotorControlDevRef"=w285) -> ("error out"=w279:errorcluster, "Motor Output"=w278:dbl, "MotorControlDevRef"=w277:T4)  [unwired: 6 in]
          n157 = call <vilib>:"WPI_MotorControlSafetyConfig.vi"("error in (no error)"=w282, "timeout (s)"=w281, "mode"=WPI_SafetyOutputConfigMenu."Enable", "MotorControlDevRef"=w280) -> ()  [unwired: 6 in, 2 out]
          n158 = call <vilib>:"WPI_MotorControlSafetyConfig.vi"("error in (no error)"=w279, "timeout (s)"=w278, "mode"=WPI_SafetyOutputConfigMenu."Enable", "MotorControlDevRef"=w277) -> ()  [unwired: 6 in, 2 out]
        }
        frame #2 {
          # "Push out \nfor 1.5 sec"
          n159 = Wait (ms)(milliseconds to wait=u32 1500) -> ()  [unwired: 1 out]
        }
        frame #3 {
          w290 = 0.0 ("t")
          # "Stop Wheels"
          n160 = Negate(x=w290) -> (-x=w291:dbl)
          n161 = call <vilib>:"WPI_MotorControlRefNum Registry Get.vi"("refnum name"="LeftWheel") -> ("error out"=w305:errorcluster, "MotorControlDevRef"=w304:T4)  [unwired: 9 in]
          n162 = call <vilib>:"WPI_MotorControlRefNum Registry Get.vi"("refnum name"="RightWheel") -> ("error out"=w303:errorcluster, "MotorControlDevRef"=w302:T4)  [unwired: 9 in]
          n163 = call <vilib>:"WPI_MotorControlSetOutput.vi"("error in (no error)"=w305, "Output"=w290, "MotorControlDevRef"=w304) -> ("error out"=w299:errorcluster, "Motor Output"=w298:dbl, "MotorControlDevRef"=w297:T4)  [unwired: 6 in]
          n164 = call <vilib>:"WPI_MotorControlSetOutput.vi"("error in (no error)"=w303, "Output"=w291, "MotorControlDevRef"=w302) -> ("error out"=w296:errorcluster, "Motor Output"=w295:dbl, "MotorControlDevRef"=w294:T4)  [unwired: 6 in]
          n165 = call <vilib>:"WPI_MotorControlSafetyConfig.vi"("error in (no error)"=w299, "timeout (s)"=w298, "mode"=WPI_SafetyOutputConfigMenu."Enable", "MotorControlDevRef"=w297) -> ()  [unwired: 6 in, 2 out]
          n166 = call <vilib>:"WPI_MotorControlSafetyConfig.vi"("error in (no error)"=w296, "timeout (s)"=w295, "mode"=WPI_SafetyOutputConfigMenu."Enable", "MotorControlDevRef"=w294) -> ()  [unwired: 6 in, 2 out]
        }
      }
    }
  }
  n167 = case shown="False" w3 {
    frame False {
      n168 = call-poly <vilib>:"SD Write Value.vi"("Boolean"=FALSE, "Name"="DB/LED 1") -> ()  [unwired: 8 in, 2 out]
    }
    frame True {
      n169 = call-poly <vilib>:"SD Write Value.vi"("Boolean"=TRUE, "Name"="DB/LED 1") -> ()  [unwired: 8 in, 2 out]
      n170 = global read "AutoVar.vi" "State"() -> (w310:string)
      n171 = case shown="\"Start\"" w310 {
        frame "False", Default {
        }
        frame "Start" {
          w312 = 1.0 ("t")
          # "Move Outer Wheels"
          # "Pull in"
          n172 = Negate(x=w312) -> (-x=w313:dbl)
          n173 = call <vilib>:"WPI_MotorControlRefNum Registry Get.vi"("refnum name"="LeftWheel") -> ("error out"=w327:errorcluster, "MotorControlDevRef"=w326:T4)  [unwired: 9 in]
          n174 = call <vilib>:"WPI_MotorControlRefNum Registry Get.vi"("refnum name"="RightWheel") -> ("error out"=w325:errorcluster, "MotorControlDevRef"=w324:T4)  [unwired: 9 in]
          n175 = call <vilib>:"WPI_MotorControlSetOutput.vi"("error in (no error)"=w327, "Output"=w312, "MotorControlDevRef"=w326) -> ("error out"=w321:errorcluster, "Motor Output"=w320:dbl, "MotorControlDevRef"=w319:T4)  [unwired: 6 in]
          n176 = global write "AutoVar.vi" "State"("Looking1" ("State")) -> ()
          n177 = call <vilib>:"WPI_MotorControlSetOutput.vi"("error in (no error)"=w325, "Output"=w313, "MotorControlDevRef"=w324) -> ("error out"=w318:errorcluster, "Motor Output"=w317:dbl, "MotorControlDevRef"=w316:T4)  [unwired: 6 in]
          n178 = call <vilib>:"WPI_MotorControlSafetyConfig.vi"("error in (no error)"=w321, "timeout (s)"=w320, "mode"=WPI_SafetyOutputConfigMenu."Enable", "MotorControlDevRef"=w319) -> ()  [unwired: 6 in, 2 out]
          n179 = call <vilib>:"WPI_MotorControlSafetyConfig.vi"("error in (no error)"=w318, "timeout (s)"=w317, "mode"=WPI_SafetyOutputConfigMenu."Enable", "MotorControlDevRef"=w316) -> ()  [unwired: 6 in, 2 out]
        }
        frame "End" {
          w328 = 0.0 ("t")
          # "Stop"
          n180 = Negate(x=w328) -> (-x=w329:dbl)
          n181 = call <vilib>:"WPI_MotorControlRefNum Registry Get.vi"("refnum name"="LeftWheel") -> ("error out"=w343:errorcluster, "MotorControlDevRef"=w342:T4)  [unwired: 9 in]
          n182 = call <vilib>:"WPI_MotorControlRefNum Registry Get.vi"("refnum name"="RightWheel") -> ("error out"=w341:errorcluster, "MotorControlDevRef"=w340:T4)  [unwired: 9 in]
          n183 = call <vilib>:"WPI_MotorControlSetOutput.vi"("error in (no error)"=w343, "Output"=w328, "MotorControlDevRef"=w342) -> ("error out"=w337:errorcluster, "Motor Output"=w336:dbl, "MotorControlDevRef"=w335:T4)  [unwired: 6 in]
          n184 = call <vilib>:"WPI_MotorControlSetOutput.vi"("error in (no error)"=w341, "Output"=w329, "MotorControlDevRef"=w340) -> ("error out"=w334:errorcluster, "Motor Output"=w333:dbl, "MotorControlDevRef"=w332:T4)  [unwired: 6 in]
          n185 = call <vilib>:"WPI_MotorControlSafetyConfig.vi"("error in (no error)"=w337, "timeout (s)"=w336, "mode"=WPI_SafetyOutputConfigMenu."Enable", "MotorControlDevRef"=w335) -> ()  [unwired: 6 in, 2 out]
          n186 = call <vilib>:"WPI_MotorControlSafetyConfig.vi"("error in (no error)"=w334, "timeout (s)"=w333, "mode"=WPI_SafetyOutputConfigMenu."Enable", "MotorControlDevRef"=w332) -> ()  [unwired: 6 in, 2 out]
        }
        frame "Looking1" {
          # "If It can't see the tote then move"
          # "Positions Robot infront of Tote"
          # "If box is Just right"
          # "If box is too far"
          n187 = global read "Global 2.vi" "Scale%"() -> (w346:dbl)
          n188 = In Range and Coerce(upper limit=100.0, x=w346, lower limit=85.0) -> (In Range?=w348:bool)  [unwired: 1 out]
          n189 = Less?(x=w346, y=100.0) -> (x < y?=w353:bool)
          n190 = Select(t=0.0, s=w348, f=0.5) -> (s? t:f=w360:dbl)
          n191 = Select(t="Looking2", s=w348, f="Looking1" ("t")) -> (s? t:f=w347:string)
          n192 = Select(t=0.5, s=w353, f=w360) -> (s? t:f=w350:dbl)
          n193 = global write "AutoVar.vi" "State"(w347) -> ()
          n194 = global write "AutoVar.vi" "Scale at that point"(w346) -> ()
          n195 = call <vilib>:"WPI_RobotDriveRefNum Registry Get.vi"("refnum name"="Left and Right Motors") -> ("RobotDriveDevRef"=w356:T13)  [unwired: 1 in, 9 out]
          n196 = call-poly <vilib>:"WPI_RobotDriveArcadeDrive.vi"("Y axis value"=w350, "RobotDriveDevRef"=w356) -> ("Motor Values"=w355:dbl[], "RobotDriveDevRef"=w359:T13)  [unwired: 2 in, 6 out]
          n197 = call-poly <vilib>:"SD Write Value.vi"("Numeric Array"=w355, "Name"="RobotDrive Motors") -> ()  [unwired: 8 in, 2 out]
          n198 = call <vilib>:"WPI_RobotDriveDelayAndUpdateSafety.vi"("Delay (s)"=1.0, "RobotDriveDevRef"=w359) -> ()  [unwired: 8 in, 2 out]
        }
        frame "Looking2" {
          # "If It can't see the tote then move"
          # "Positions Robot infront of Tote"
          # "If box is Just right"
          n199 = global read "Global 2.vi" "Scale%"() -> (w372:dbl)
          n200 = In Range and Coerce(upper limit=100.0, x=w372, lower limit=85.0) -> (In Range?=w368:bool)  [unwired: 1 out]
          n201 = Select(t=1.0, s=w368, f=0.0) -> (s? t:f=w366:dbl)
          n202 = Select(t="Looking2", s=w368, f="Done" ("t")) -> (s? t:f=w367:string)
          n203 = global write "AutoVar.vi" "State"(w367) -> ()
          n204 = call <vilib>:"WPI_RobotDriveRefNum Registry Get.vi"("refnum name"="Left and Right Motors") -> ("RobotDriveDevRef"=w375:T13)  [unwired: 1 in, 9 out]
          n205 = call-poly <vilib>:"WPI_RobotDriveArcadeDrive.vi"("Y axis value"=w366, "RobotDriveDevRef"=w375) -> ("Motor Values"=w374:dbl[], "RobotDriveDevRef"=w378:T13)  [unwired: 2 in, 6 out]
          n206 = call-poly <vilib>:"SD Write Value.vi"("Numeric Array"=w374, "Name"="RobotDrive Motors") -> ()  [unwired: 8 in, 2 out]
          n207 = call <vilib>:"WPI_RobotDriveDelayAndUpdateSafety.vi"("Delay (s)"=1.0, "RobotDriveDevRef"=w378) -> ()  [unwired: 8 in, 2 out]
        }
        frame "Done" {
          w381 = "RobotDrive Motors" ("Name")
          w392 = 0.0 ("t")
          # "drive back"
          # "Turn 90 degrees"
          # "Stop Outer Wheels"
          n208 = Negate(x=w392) -> (-x=w393:dbl)
          n209 = call <vilib>:"WPI_MotorControlRefNum Registry Get.vi"("refnum name"="LeftWheel") -> ("error out"=w407:errorcluster, "MotorControlDevRef"=w406:T4)  [unwired: 9 in]
          n210 = call <vilib>:"WPI_MotorControlRefNum Registry Get.vi"("refnum name"="RightWheel") -> ("error out"=w405:errorcluster, "MotorControlDevRef"=w404:T4)  [unwired: 9 in]
          n211 = call <vilib>:"WPI_MotorControlSetOutput.vi"("error in (no error)"=w407, "Output"=w392, "MotorControlDevRef"=w406) -> ("error out"=w401:errorcluster, "Motor Output"=w400:dbl, "MotorControlDevRef"=w399:T4)  [unwired: 6 in]
          n212 = call <vilib>:"WPI_MotorControlSetOutput.vi"("error in (no error)"=w405, "Output"=w393, "MotorControlDevRef"=w404) -> ("error out"=w398:errorcluster, "Motor Output"=w397:dbl, "MotorControlDevRef"=w396:T4)  [unwired: 6 in]
          n213 = call <vilib>:"WPI_MotorControlSafetyConfig.vi"("error in (no error)"=w401, "timeout (s)"=w400, "mode"=WPI_SafetyOutputConfigMenu."Enable", "MotorControlDevRef"=w399) -> ()  [unwired: 6 in, 2 out]
          n214 = call <vilib>:"WPI_MotorControlSafetyConfig.vi"("error in (no error)"=w398, "timeout (s)"=w397, "mode"=WPI_SafetyOutputConfigMenu."Enable", "MotorControlDevRef"=w396) -> ()  [unwired: 6 in, 2 out]
          n215 = call <vilib>:"WPI_RobotDriveRefNum Registry Get.vi"("refnum name"="Left and Right Motors") -> ("RobotDriveDevRef"=w384:T13)  [unwired: 1 in, 9 out]
          n216 = call-poly <vilib>:"WPI_RobotDriveArcadeDrive.vi"("X axis value"=0.7, "RobotDriveDevRef"=w384) -> ("Motor Values"=w383:dbl[], "RobotDriveDevRef"=w390:T13)  [unwired: 2 in, 6 out]
          n217 = call-poly <vilib>:"SD Write Value.vi"("Numeric Array"=w383, "Name"=w381) -> ()  [unwired: 8 in, 2 out]
          n218 = call <vilib>:"WPI_RobotDriveDelayAndUpdateSafety.vi"("Delay (s)"=0.3, "RobotDriveDevRef"=w390) -> ("RobotDriveDevRef 2"=w389:T13)  [unwired: 8 in, 1 out]
          n219 = call-poly <vilib>:"WPI_RobotDriveArcadeDrive.vi"("Y axis value"=-0.7 ("X axis value"), "RobotDriveDevRef"=w389) -> ("Motor Values"=w382:dbl[], "RobotDriveDevRef"=w388:T13)  [unwired: 2 in, 6 out]
          n220 = call-poly <vilib>:"SD Write Value.vi"("Numeric Array"=w382, "Name"=w381) -> ()  [unwired: 8 in, 2 out]
          n221 = call <vilib>:"WPI_RobotDriveDelayAndUpdateSafety.vi"("Delay (s)"=1.3, "RobotDriveDevRef"=w388) -> ()  [unwired: 8 in, 2 out]
        }
      }
    }
  }
  n222 = disable-structure shown="Disabled" {
    frame Disabled {
      # "Carry green bin"
      n223 = flat-sequence {
        tunnel: [w415] -> w413
        tunnel: [w414] -> w412
        tunnel: w413 -> [w425]
        tunnel: w412 -> [w424]
        tunnel: [w428] -> w411
        tunnel: [w427] -> w410
        tunnel: w411 -> [w438]
        tunnel: w410 -> [w437]
        tunnel: [w441] -> w409
        tunnel: [w440] -> w408
        tunnel: w409 -> [w451]
        tunnel: w408 -> [w450]
        frame #0 {
          w417 = -0.7 ("Output")
          # "zero actuators before moving"
          # "Wait for 1.5 seconds"
          n224 = call <vilib>:"WPI_MotorControlRefNum Registry Get.vi"("refnum name"="Linear Actuator1") -> ("error out"=w420:errorcluster, "MotorControlDevRef"=w419:T4)  [unwired: 9 in]
          n225 = call <vilib>:"WPI_MotorControlRefNum Registry Get.vi"("refnum name"="Linear Actuator0") -> ("error out"=w423:errorcluster, "MotorControlDevRef"=w422:T4)  [unwired: 9 in]
          n226 = call <vilib>:"WPI_MotorControlSetOutput.vi"("error in (no error)"=w420, "Output"=w417, "MotorControlDevRef"=w419) -> ("MotorControlDevRef"=w414:T4)  [unwired: 6 in, 2 out]
          n227 = call <vilib>:"WPI_MotorControlSetOutput.vi"("error in (no error)"=w423, "Output"=w417, "MotorControlDevRef"=w422) -> ("MotorControlDevRef"=w415:T4)  [unwired: 6 in, 2 out]
          n228 = Wait (ms)(milliseconds to wait=u32 1500) -> ()  [unwired: 1 out]
        }
        frame #1 {
          w426 = 0.0 ("Output")
          n229 = call <vilib>:"WPI_MotorControlSetOutput.vi"("Output"=w426, "MotorControlDevRef"=w424) -> ()  [unwired: 7 in, 3 out]
          n230 = call <vilib>:"WPI_MotorControlSetOutput.vi"("Output"=w426, "MotorControlDevRef"=w425) -> ()  [unwired: 7 in, 3 out]
        }
        frame #2 {
          w430 = 0.7 ("Output")
          # "Move actuators up to a particular position first"
          # "Time to wait is not yet known\nbut for now its 0.3sec"
          n231 = call <vilib>:"WPI_MotorControlRefNum Registry Get.vi"("refnum name"="Linear Actuator1") -> ("error out"=w433:errorcluster, "MotorControlDevRef"=w432:T4)  [unwired: 9 in]
          n232 = call <vilib>:"WPI_MotorControlRefNum Registry Get.vi"("refnum name"="Linear Actuator0") -> ("error out"=w436:errorcluster, "MotorControlDevRef"=w435:T4)  [unwired: 9 in]
          n233 = call <vilib>:"WPI_MotorControlSetOutput.vi"("error in (no error)"=w433, "Output"=w430, "MotorControlDevRef"=w432) -> ("MotorControlDevRef"=w427:T4)  [unwired: 6 in, 2 out]
          n234 = call <vilib>:"WPI_MotorControlSetOutput.vi"("error in (no error)"=w436, "Output"=w430, "MotorControlDevRef"=w435) -> ("MotorControlDevRef"=w428:T4)  [unwired: 6 in, 2 out]
          n235 = Wait (ms)(milliseconds to wait=u32 300) -> ()  [unwired: 1 out]
        }
        frame #3 {
          w439 = 0.0 ("Output")
          n236 = call <vilib>:"WPI_MotorControlSetOutput.vi"("Output"=w439, "MotorControlDevRef"=w437) -> ()  [unwired: 7 in, 3 out]
          n237 = call <vilib>:"WPI_MotorControlSetOutput.vi"("Output"=w439, "MotorControlDevRef"=w438) -> ()  [unwired: 7 in, 3 out]
        }
        frame #4 {
          w443 = -0.7 ("Output")
          # "Move actuators up to carry up the green bin"
          # "One second should be enough.."
          n238 = call <vilib>:"WPI_MotorControlRefNum Registry Get.vi"("refnum name"="Linear Actuator1") -> ("error out"=w446:errorcluster, "MotorControlDevRef"=w445:T4)  [unwired: 9 in]
          n239 = call <vilib>:"WPI_MotorControlRefNum Registry Get.vi"("refnum name"="Linear Actuator0") -> ("error out"=w449:errorcluster, "MotorControlDevRef"=w448:T4)  [unwired: 9 in]
          n240 = call <vilib>:"WPI_MotorControlSetOutput.vi"("error in (no error)"=w446, "Output"=w443, "MotorControlDevRef"=w445) -> ("MotorControlDevRef"=w440:T4)  [unwired: 6 in, 2 out]
          n241 = call <vilib>:"WPI_MotorControlSetOutput.vi"("error in (no error)"=w449, "Output"=w443, "MotorControlDevRef"=w448) -> ("MotorControlDevRef"=w441:T4)  [unwired: 6 in, 2 out]
          n242 = Wait (ms)(milliseconds to wait=u32 1000) -> ()  [unwired: 1 out]
        }
        frame #5 {
          w452 = 0.0 ("Output")
          n243 = call <vilib>:"WPI_MotorControlSetOutput.vi"("Output"=w452, "MotorControlDevRef"=w450) -> ()  [unwired: 7 in, 3 out]
          n244 = call <vilib>:"WPI_MotorControlSetOutput.vi"("Output"=w452, "MotorControlDevRef"=w451) -> ()  [unwired: 7 in, 3 out]
        }
      }
    }
    frame Enabled {
    }
  }
